vi "test_TCP_Open connection using Initialize node.vi"(8 "error in (no error)":errorcluster, 11 "TestCase in":refnum<class "Ethernet Protocol Tests.lvclass">) -> (0 "error out":errorcluster, 3 "TestCase out":refnum<class "Ethernet Protocol Tests.lvclass">)   [LabVIEW 2019, in "Ethernet Protocol Tests.lvclass"]
uses:
  Ethernet Protocol Tests.lvclass
  TCP/TCP.lvclass
  TCP/TCP.lvclass/TCP.ctl
  <vilib>/addons/_JKI Toolkits/VI Tester/TestCase.llb/TestCase.lvclass
  C:/Program Files (x86)/National Instruments/LabVIEW 2019/vi.lib/addons/_JKI Toolkits/VI Tester/TestCase.llb/TestCase.lvclass
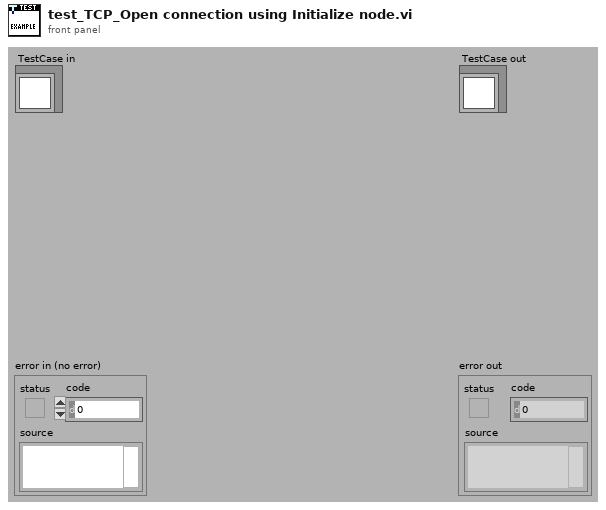
[diagram p1: front panel]
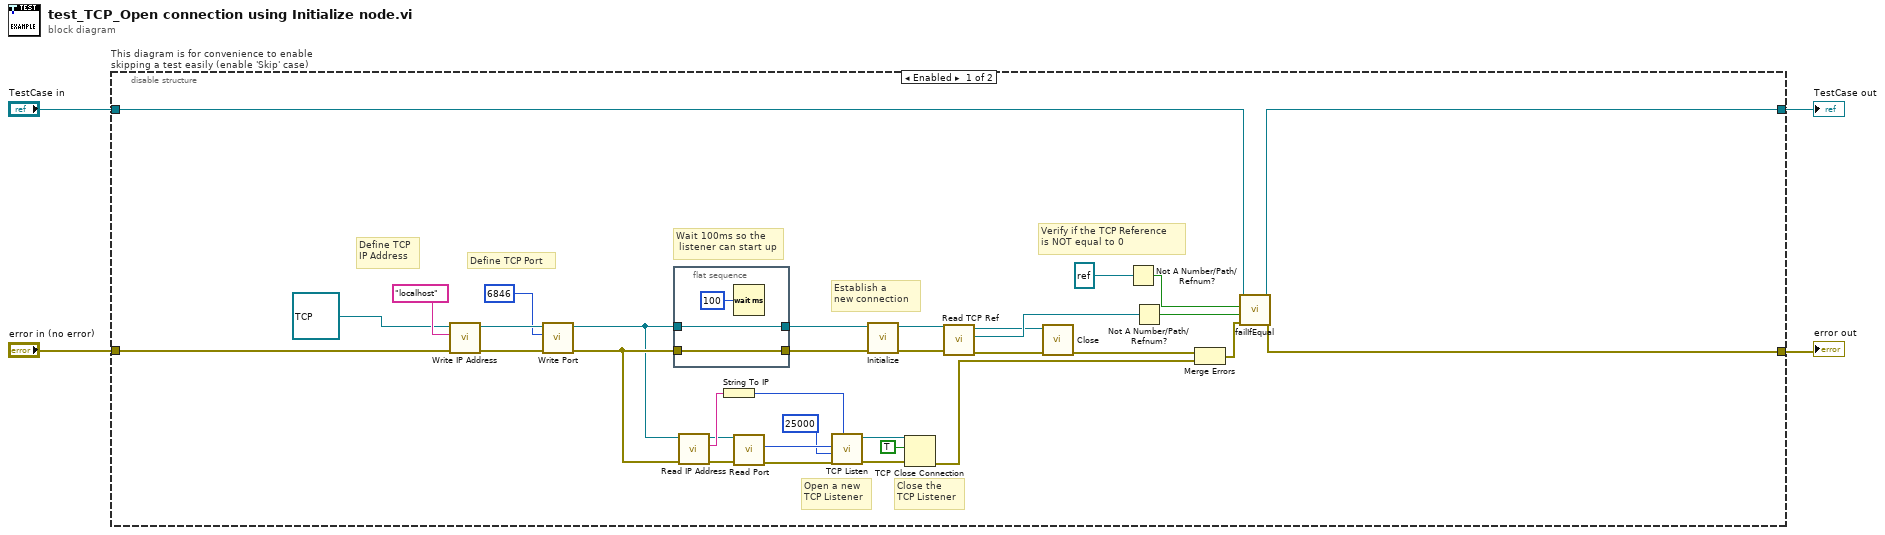
[diagram p0: block diagram]
diagram:
  n1 = disable-structure "This diagram is for convenience to enable skipping a test easily (enable 'Skip' case)" shown="Enabled" {
    disable-tunnel: "TestCase in" -> [w38 w45]
    disable-tunnel: [w19 w43] -> w1
    disable-tunnel: [w18 w44] -> w3
    disable-tunnel: "error in (no error)" -> [w32 w42]
    frame Enabled {
      # "Wait 100ms so the\n listener can start up"
      # "Verify if the TCP Reference \nis NOT equal to 0"
      # "Close the \nTCP Listener"
      # "Open a new \nTCP Listener"
      # "Establish a \nnew connection"
      # "Define TCP Port"
      # "Define TCP\nIP Address"
      n2 = call "Write IP Address.vi"("error in (no error)"=w32, "IP Address"="localhost", "Ethernet in"=refnum<class "TCP.lvclass"> refnum ("Protocols.lvlib:TCP.lvclass")) -> ("error out"=w35:errorcluster, "Ethernet out"=w36:refnum<class "TCP.lvclass">)  [unwired: 7 in]
      n3 = call "Write Port.vi"("error in (no error)"=w35, "Port"=u16 6846, "Ethernet in"=w36) -> ("error out"=w7:errorcluster, "Ethernet out"=w6:refnum<class "TCP.lvclass">)  [unwired: 7 in]
      n4 = flat-sequence {
        tunnel: w7 -> [w40]
        tunnel: [w40] -> w10
        tunnel: w6 -> [w39]
        tunnel: [w39] -> w8
        frame #0 {
          n5 = Wait (ms)(milliseconds to wait=u32 100) -> ()  [unwired: 1 out]
        }
      }
      n6 = call "Read IP Address.vi"("error in (no error)"=w7, "Ethernet in"=w6) -> ("error out"=w29:errorcluster, "IP Address"=w31:string, "Ethernet out"=w28:refnum<class "TCP.lvclass">)  [unwired: 7 in]
      n7 = String To IP(1:w31) -> (0:w30:u32)
      n8 = call "Read Port.vi"("error in (no error)"=w29, "Ethernet in"=w28) -> ("error out"=w27:errorcluster, "Port"=w26:u16)  [unwired: 7 in, 1 out]
      n9 = call <vilib>:"TCP Listen.vi"("net address"=w30, "error in (no error)"=w27, "timeout ms (wait forever: -1)"=25000, "port"=w26) -> ("error out"=w24:errorcluster, "connection ID"=w23:refnum<k5>)  [unwired: 3 in, 3 out]
      n10 = call-dynamic "Initialize.vi"("error in (no error)"=w10, "Ethernet in"=w8) -> ("error out"=w9:errorcluster, "Ethernet out"=w5:refnum<class "TCP.lvclass">)  [unwired: 8 in]
      n11 = TCP Close Connection(connection ID=w23, abort (F)=TRUE, error in (no error)=w24) -> (error out=w21:errorcluster)  [unwired: 1 out]
      n12 = call "Read TCP Ref.vi"("error in (no error)"=w9, "Ethernet in"=w5) -> ("error out"=w13:errorcluster, "TCP Ref"=w17:refnum<k5>, "Ethernet out"=w11:refnum<class "TCP.lvclass">)  [unwired: 7 in]
      n13 = call-dynamic "Close.vi"("error in (no error)"=w13, "Ethernet in"=w11) -> ("error out"=w12:errorcluster)  [unwired: 8 in, 1 out]
      n14 = Not A Number/Path/Refnum?(number/path/refnum=refnum<k5> refnum ("TCP Ref")) -> (NaN/Path/Refnum?=w14:bool)
      n15 = Not A Number/Path/Refnum?(number/path/refnum=w17) -> (NaN/Path/Refnum?=w16:bool)
      n16 = Merge Errors(w12, w21) -> (w20:errorcluster)
      n17 = call-dynamic "failIfEqual.vi"("error in (no error)"=w20, "y"=w16, "x"=w14, "TestCase in"=w38) -> ("error out"=w18:errorcluster, "TestCase out"=w19:refnum<class "Ethernet Protocol Tests.lvclass">)  [unwired: 6 in]
    }
    frame Disabled {
      # "skip test result while test is under development"
      n18 = call <vilib>:"skip.vi"("error in (no error)"=w42, "TestCase in"=w45) -> ("error out"=w44:errorcluster, "TestCase out"=w43:refnum<class "Ethernet Protocol Tests.lvclass">)  [unwired: 8 in]
    }
  }
  "error out" <- w3
  "TestCase out" <- w1
